vi "Set Goal Accel.vi"(0 "VISA resource name":refnum<visa-resource-name>, 5 "Motor ID (0)":u8, 7 "Goal Accel. (Degree/s^2)":dbl=150.0, 11 "error in (no error)":errorcluster) -> (4 "VISA resource name out":refnum<visa-resource-name>, 15 "error out":errorcluster)   [LabVIEW 2016, in "Dynamixel Motor.lvlib"]
doc: "Sets the goal acceleration for the motor."
uses:
  Dynamixel Motor.lvlib
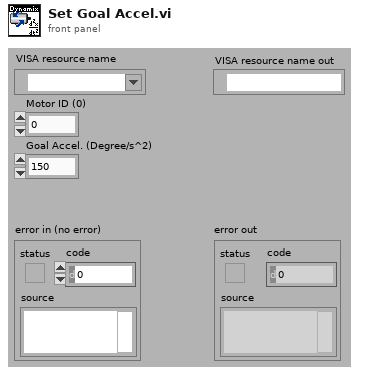
[diagram p1: front panel]
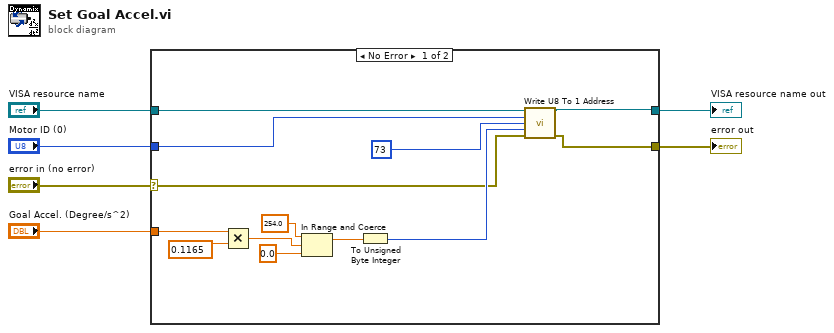
[diagram p0: block diagram]
diagram:
  n1 = case shown="No Error" "error in (no error)" {
    selector: "error in (no error)" -> [w8 w21]
    tunnel: "VISA resource name" -> [w12 w20]
    tunnel: [w13 w20] -> w5
    tunnel: [w11 w21] -> w4
    tunnel: "Motor ID (0)" -> [w7 _]
    tunnel: "Goal Accel. (Degree/s^2)" -> [w18 _]
    frame No Error {
      n2 = Multiply(x=w18, y=0.1165) -> (x*y=w14:dbl)
      n3 = In Range and Coerce(upper limit=254.0, x=w14, lower limit=0.0) -> (coerced(x)=w15:dbl)  [unwired: 1 out]
      n4 = To Unsigned Byte Integer(number=w15) -> (unsigned 8bit integer=w9:u8)
      n5 = call "Write U8 To 1 Address.vi"("VISA resource name"=w12, "Motor ID (0)"=w7, "Address number (0)"=u8 73 ("Address"), "Parameter (0)"=w9, "error in (no error)"=w8) -> ("VISA resource name out"=w13:refnum<visa-resource-name>, "error out"=w11:errorcluster)  [unwired: 9 in]
    }
    frame Error {
    }
  }
  "VISA resource name out" <- w5
  "error out" <- w4
